vi "MGCC_LoadFcst.vi"(1 "InputTimeSeries":dbl[](array[numeric])) -> (0 "OutputTimeSeries":dbl[](array[numeric]))   [LabVIEW 2016]
doc: "-----------------------------------------------------------------------------------------------------------------------\nCopyright <2019> <The University of Tennessee at Knoxville and the University of Tennessee Research Foundation>\nThis software is released under BSD-3 \nhttps://opensource.org/licenses/BSD-3-Clause \nAdditional license options available at https://utrf.tennessee.edu/industry/sample-agreements/\n-----------------------------------------------------------------------------------------------------------------------\n\nThis VI realizes the load forecasting function in the MGCC. Input is a historical time series of load data in 15 min intervals. Output is 96-point-ahead (24 hrs) of the load. This VI uses a simple AR model for forecasting."
uses:
  <vilib>/addons/Time Series Analysis/Modeling and Prediction.llb/TSA AR Modeling Order (Array).vi
  <vilib>/addons/Time Series Analysis/Modeling and Prediction.llb/TSA ARMA Modeling (Array).vi
  <vilib>/addons/Time Series Analysis/Modeling and Prediction.llb/TSA ARMA Prediction (Array).vi
  <vilib>/addons/_Advanced Signal Processing/NI_AdvSigProcTSA.lvlib
panel:
  out "standard deviation":dbl[](array[numeric]) format="%.4f"
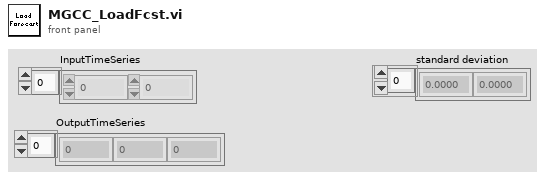
[diagram p1: front panel]
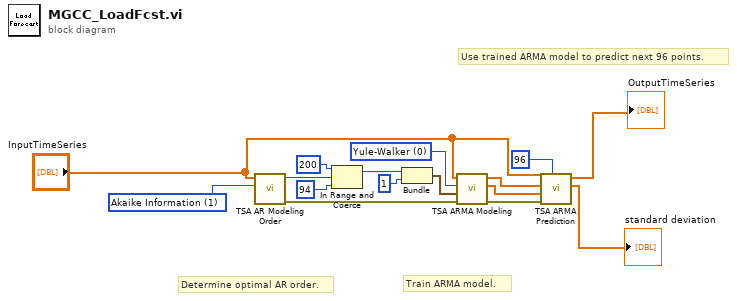
[diagram p0: block diagram]
diagram:
  w8 = 1 items=["Final Prediction Error"=0, "Akaike Information"=1, "Bayesian Information"=4, "Minimal Description Length"=2, "Phi Criterion"=3, "-"=-1, "Partial Correlation Function"=6] ("method")
  w9 = u16 0 items=["Yule-Walker", "High order AR", "Polynomial"] ("method")
  # "Use trained ARMA model to predict next 96 points."
  # "Train ARMA model."
  # "Determine optimal AR order."
  n1 = call-poly <vilib>:"TSA AR Modeling Order.vi"("method"=w8, "Xt"="InputTimeSeries") -> ("error out"=w7:errorcluster, "optimal AR order"=w4:i32)  [unwired: 7 in, 1 out]
  n2 = In Range and Coerce(upper limit=200, x=w4, lower limit=94) -> (coerced(x)=w1:i32)  [unwired: 1 out]
  n3 = Bundle("upper limit"=w1, 1) -> (w5:cluster{"upper limit":i32, i32})  [unwired: 1 in]
  n4 = call-poly <vilib>:"TSA ARMA Modeling.vi"("error in (no error)"=w7, "ARMA order"=w5, "method"=w9, "Xt"="InputTimeSeries") -> ("error out"=w12:errorcluster, "MA coefficients"=w10:dbl[], "AR coefficients"=w11:dbl[])  [unwired: 4 in, 1 out]
  n5 = call-poly <vilib>:"TSA ARMA Prediction.vi"("number of points"=96, "error in (no error)"=w12, "MA coefficients"=w10, "AR coefficients"=w11, "Xt"="InputTimeSeries") -> ("standard deviation"=→"standard deviation":dbl[], "predicted series"=→"OutputTimeSeries":dbl[])  [unwired: 4 in, 1 out]
